vi "Save-Recall Setup.vi"(8 "error in (no error)":errorcluster, 9 "Memory Location (1: Location 1)":u16(ring)=1 items=["Location 1"=1, "Location 2"=2, "Location 3"=3, "Location 4"=4, "Location 5"=5, "Location 6"=6, "Location 7"=7, "Location 8"=8, "Location 9"=9, "Location 10"=10], 10 "Operation (0: Save)":u16(ring) items=["Save", "Recall"], 11 "VISA resource name":refnum<visa-resource-name>) -> (0 "error out":errorcluster, 3 "VISA resource name out":refnum<visa-resource-name>)   [LabVIEW 2017, in "Scope.lvlib" / "Tektronix DPO MSO 2000 4000 Series.lvlib"]
doc: "Saves instruments settings to the selected memory location or recalls instrument settings from the selected memory location."
uses:
  Tektronix DPO MSO 2000 4000 Series.lvlib
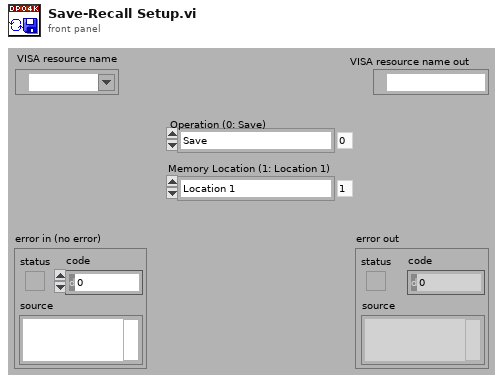
[diagram p1: front panel]
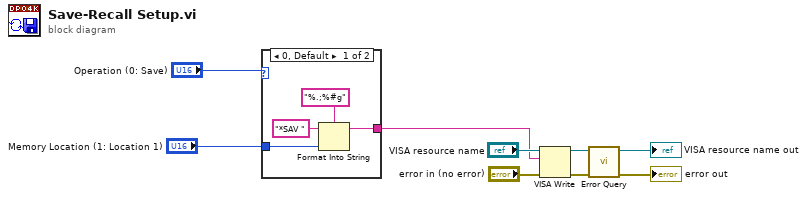
[diagram p0: block diagram]
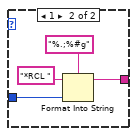
[diagram p2: hidden frame]
diagram:
  n1 = case shown="0, Default" "Operation (0: Save)" {
    tunnel: "Memory Location (1: Location 1)" -> [w13 w15]
    tunnel: [w10 w14] -> w5
    frame 0, Default {
      n2 = Format Into String(format string="%.;%#g", initial string="*SAV ", w13) -> (resulting string=w10:string)  [unwired: 1 in, 1 out]
    }
    frame 1 {
      n3 = Format Into String(format string="%.;%#g", initial string="*RCL ", w15) -> (resulting string=w14:string)  [unwired: 1 in, 1 out]
    }
  }
  n4 = VISA Write(VISA resource name="VISA resource name", write buffer=w5, error in (no error)="error in (no error)") -> (VISA resource name out=w4:refnum<visa-resource-name>, error out=w3:errorcluster)  [unwired: 1 out]
  n5 = call "Error Query.vi"("error in (no error)"=w3, "VISA resource name"=w4) -> ("error out"=→"error out":errorcluster, "VISA resource name out"=→"VISA resource name out":refnum<visa-resource-name>)  [unwired: 6 in, 2 out]
